vi "Check if Computer is on AC Power.vi"(8 "error in (no error)":errorcluster) -> (0 "error out":errorcluster, 2 "AC Power?":bool)   [LabVIEW 2018]
doc: "Calls kernel32.dll GetSystemPowerStatus. If ACLineStatus is 1 (PC is running off AC power), AC Power? is true.\n\nVI by Pulido Technologies LLC"
uses:
  kernel32.dll
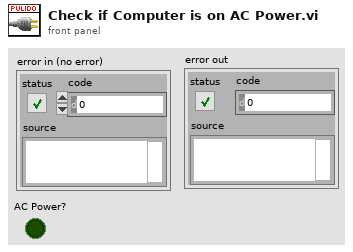
[diagram p1: front panel]
types:
  T1 = cluster{"ACLineStatus":u8, "BatteryFlag":u8, "BaterryLifePercent":u8, "Reserved":u8, "BatteryLifeTime":i32, "BatteryFullLifeTime":i32}
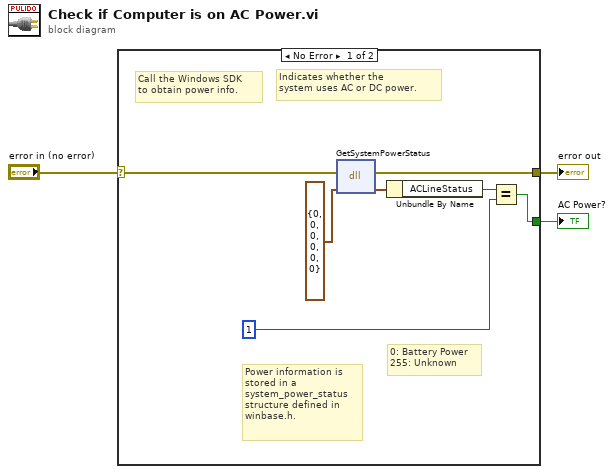
[diagram p0: block diagram]
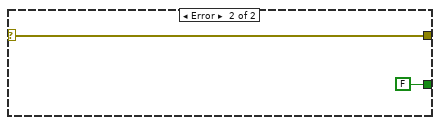
[diagram p2: hidden frame]
diagram:
  n1 = case shown="No Error" "error in (no error)" {
    selector: "error in (no error)" -> [w7 w12]
    tunnel: [w8 FALSE] -> w3
    tunnel: [w5 w12] -> w1
    frame No Error {
      # "0: Battery Power\n255: Unknown"
      # "Power information is\nstored in a\nsystem_power_status\nstructure defined in\nwinbase.h."
      # "Indicates whether the\nsystem uses AC or DC power."
      # "Call the Windows SDK\nto obtain power info."
      n2 = dll-call lib="kernel32.dll" fn="GetSystemPowerStatus"(error in=w7, "system_power_status"=T1 {"ACLineStatus"=0, "BatteryFlag"=0, "BaterryLifePercent"=0, "Reserved"=0, "BatteryLifeTime"=0, "BatteryFullLifeTime"=0}) -> (error out=w5:errorcluster, "system_power_status"=w6:T1)  [unwired: 3 in, 1 out]
      n3 = Unbundle By Name(w6) -> ("ACLineStatus"=w4:u8)
      n4 = Equal?(x=w4, y=u8 1) -> (x = y?=w8:bool)
    }
    frame Error {
    }
  }
  "AC Power?" <- w3
  "error out" <- w1
